vi "Logger_Init.vi"(6 "Group Config":T1[](array[typedef]), 7 "Log To Computer?":bool, 8 "Logging Settings":T4={"Data Grab Period"=20.0, "File Write Period"=1000.0, "Max Stored Size"=100.0, "Burst Size"=75.0}, 9 "Log To USB?":bool, 10 "File Name":string, 11 "Logger Name":string) -> (3 "TDMS DevRef Out":T3)   [LabVIEW 2016]
uses:
  <userlib>/836-Library/System/TDMS_V2/Support/Logging_Settings.ctl
  <userlib>/836-Library/System/TDMS_V2/Support/TDMS_DevRef.ctl
  <userlib>/836-Library/System/TDMS_V2/Support/Group_FIFO_Config.ctl
  <userlib>/836-Library/System/TDMS_V2/Support/Channel_FIFO_Config.ctl
  <userlib>/836-Library/System/TDMS_V2/Support/Group_Config.ctl
  <userlib>/836-Library/System/TDMS_V2/Support/Channel_Config.ctl
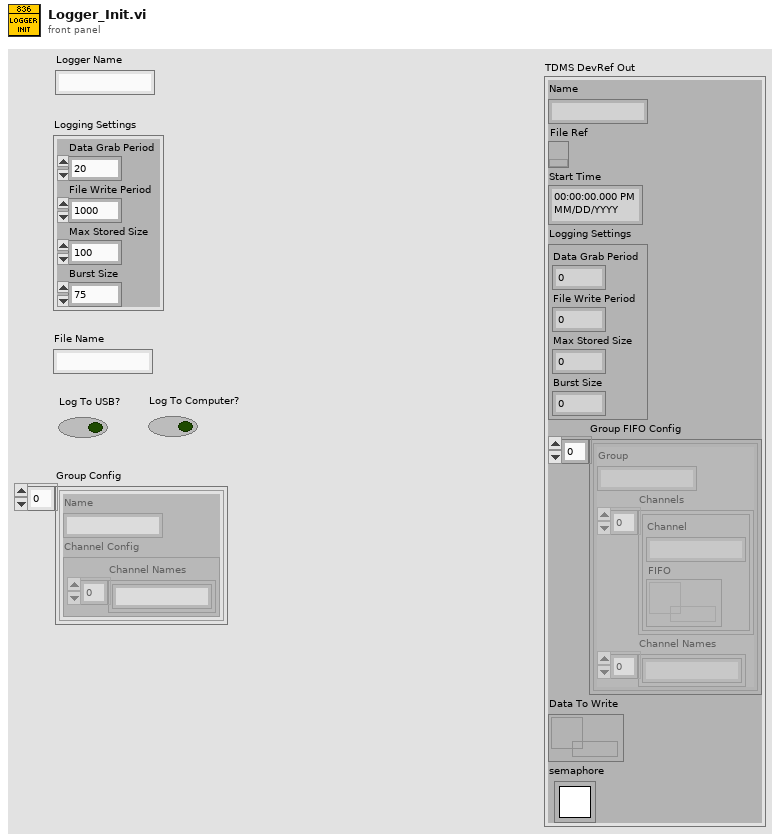
[diagram p1: front panel]
types:
  T1 = typedef "Group_Config.ctl" = cluster{"Name":string, "Channel Config":T2}
  T2 = typedef "Channel_Config.ctl" = cluster{"Channel Names":string[]}
  T3 = typedef "TDMS_DevRef.ctl" = cluster{"Name":string, "File Ref":refnum<k34>, "Start Time":timestamp, "Logging Settings":T4, "Group FIFO Config":T5[], "Data To Write":refnum<data-value>, "semaphore":T7}
  T4 = typedef "Logging_Settings.ctl" = cluster{"Data Grab Period":dbl, "File Write Period":dbl, "Max Stored Size":dbl, "Burst Size":dbl}
  T5 = typedef "Group_FIFO_Config.ctl" = cluster{"Group":string, "Channels":T6[], "Channel Names":string[]}
  T6 = typedef "Channel_FIFO_Config.ctl" = cluster{"Channel":string, "FIFO":refnum<k33>}
  T7 = typedef "Semaphore RefNum" = refnum<k1>
  T8 = enum16{"open", "open or create", "create or replace", "create", "open (read-only)"}
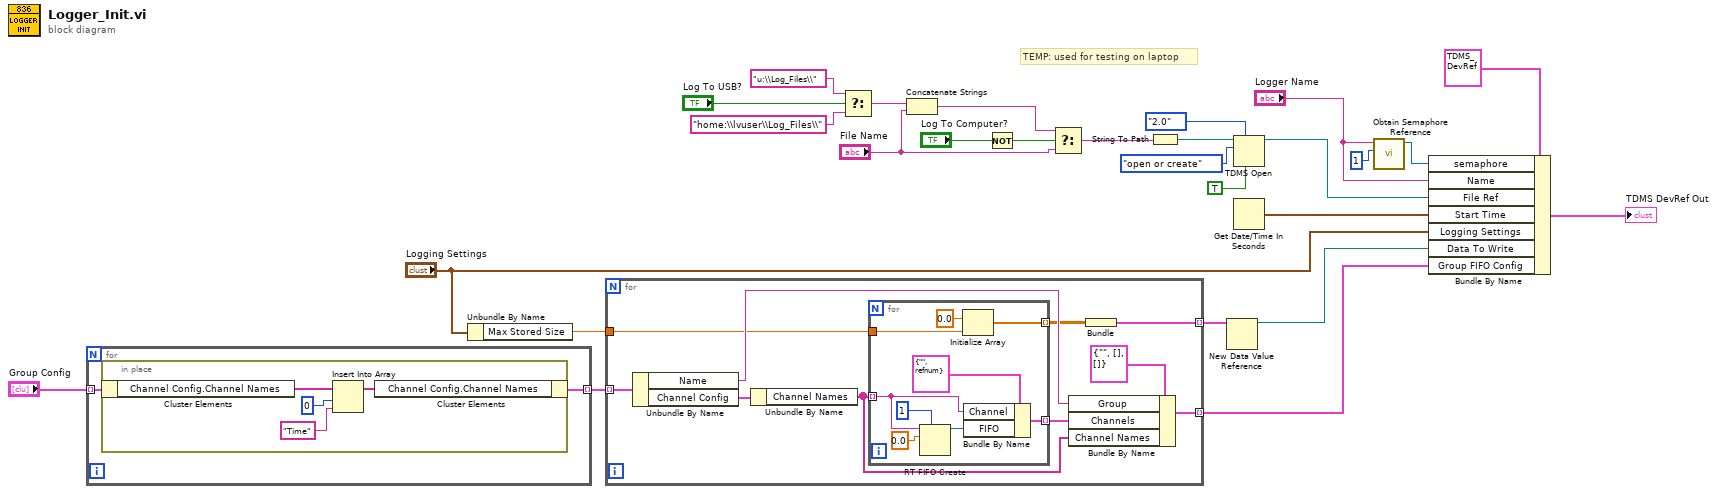
[diagram p0: block diagram]
diagram:
  # "TEMP: used for testing on laptop"
  n1 = for {
    tunnel: "Group Config" -> [w29] mode=indexing
    tunnel: [w28] -> w11 mode=indexing
    n2 = in-place {
      n3 = in-place-cluster #1(w29) -> ("Channel Config.Channel Names"=w30:string[])
      n4 = Insert Into Array(array=w30, index=0, new element="Time" ("new element/subarray")) -> (w31:string[])
      n5 = in-place-cluster #1("Channel Config.Channel Names"=w31) -> (w28:T1)
    }
  }
  n6 = Unbundle By Name("Logging Settings") -> ("Max Stored Size"=w8:dbl)
  n7 = for {
    tunnel: w11 -> [w38] mode=indexing
    tunnel: [w39] -> w17 mode=indexing
    tunnel: w8 -> [w36]
    tunnel: [w34] -> w7 mode=indexing
    n8 = Unbundle By Name(w38) -> ("Name"=w40:string, "Channel Config"=w43:T2)
    n9 = Unbundle By Name(w43) -> ("Channel Names"=w37:string[])
    n10 = for {
      tunnel: w37 -> [w48] mode=indexing
      tunnel: [w47] -> w41 mode=indexing
      tunnel: w36 -> [w46]
      tunnel: [w44] -> w35 mode=indexing
      n11 = RT FIFO Create(0:w48, 1:0.0, 4:u32 1 ("size (10)")) -> (8:w49:refnum<k33>)  [unwired: 5 in, 2 out]
      n12 = Initialize Array(0.0 ("element"), w46) -> (w44:dbl[])
      n13 = Bundle By Name(cluster=T6 {"Channel"="", "FIFO"=refnum} ("Channel Info"), "Channel"=w48, "FIFO"=w49) -> (w47:T6)
    }
    n14 = Bundle By Name(cluster=T5 {"Group"="", "Channels"=[], "Channel Names"=[]} ("Fifo Configuration"), "Group"=w40, "Channels"=w41, "Channel Names"=w37) -> (w39:T5)
    n15 = Bundle(w35) -> (w34:cluster{dbl[][]})  [unwired: 1 in]
  }
  n16 = Select(t="u:\\Log_Files\\", s="Log To USB?", f="home:\\lvuser\\Log_Files\\") -> (s? t:f=w6:string)
  n17 = Concatenate Strings(w6, "File Name") -> (w5:string)
  n18 = Not(x="Log To Computer?") -> (.not. x?=w1:bool)
  n19 = Select(t=w5, s=w1, f="File Name") -> (s? t:f=w4:string)
  n20 = String To Path(string=w4) -> (path=w24:path)
  n21 = New Data Value Reference(data value=w7) -> (data value reference=w16:refnum<data-value>)  [unwired: 1 in, 1 out]
  n22 = TDMS Open(6:TRUE ("disable buffering? (T)"), 7:enum16{"1.0", "2.0"}."2.0" ("file format version (2.0)"), 10:T8."open or create" ("operation (0:open)"), 11:w24) -> (3:w20:refnum<k34>)  [unwired: 3 in, 1 out]
  n23 = Get Date/Time In Seconds() -> (seconds since 1Jan1904=w27:timestamp)
  n24 = call <vilib>:"Obtain Semaphore Reference.vi"("size (1)"=1, "name (unnamed)"="Logger Name") -> ("semaphore"=w13:T7)  [unwired: 3 in, 2 out]
  n25 = Bundle By Name(cluster=T3 {"Name"="", "File Ref"=refnum, "Start Time"=timestamp(0 s since 1904-01-01), "Logging Settings"={"Data Grab Period"=0.0, "File Write Period"=0.0, "Max Stored Size"=0.0, "Burst Size"=0.0}, "Group FIFO Config"=[], "Data To Write"=refnum, "semaphore"=refnum}, "semaphore"=w13, "Name"="Logger Name", "File Ref"=w20, "Start Time"=w27, "Logging Settings"="Logging Settings", "Data To Write"=w16, "Group FIFO Config"=w17) -> (→"TDMS DevRef Out":T3)
